vi "getpsi.vi"() -> (3 "function return":dbl)   [LabVIEW 2019, in "HapticSTM.lvlib"]
doc: "extern \"C\" __declspec(dllexport) double getpsi();"
uses:
  HapticSTM.lvlib
  <userlib>/HapticSTM/HapticSTM.dll
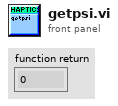
[diagram p1: front panel]
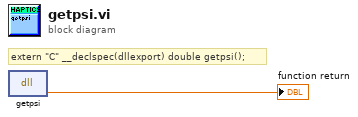
[diagram p0: block diagram]
diagram:
  # "extern \"C\" __declspec(dllexport) double getpsi();"
  n1 = dll-call lib="C:/Program Files/National Instruments/LabVIEW 2019/user.lib/HapticSTM/HapticSTM.*" fn="getpsi"() -> (→"function return":dbl)  [unwired: 3 in, 2 out]
